vi "2foldstretch.vi"() -> ()   [LabVIEW 2012]
doc: "SciScan 1.2 160622"
uses:
  GFG/GFGImageRefsGet.vi
  <vilib>/vision/NI_Vision_Development_Module.lvlib
  GFG/GFG library.lvlib
panel:
  in  "stop":bool
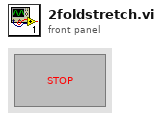
[diagram p1: front panel]
types:
  T1 = typedef "Image Type" = u32
  T2 = typedef "IMAQ Image.ctl" = refnum<image>
  T3 = cluster{"Channel 1 small":T2, "Channel 2 small":T2, "Channel 3 small":T2, "Channel 4 small":T2, "Channel 1 large":T2, "Channel 2 large":T2, "Channel 3 large":T2, "Channel 4 large":T2, "RGB overlay":T2, "ROI Image display":T2, "arb line scan display":T2, "Channel 5 large":T2}
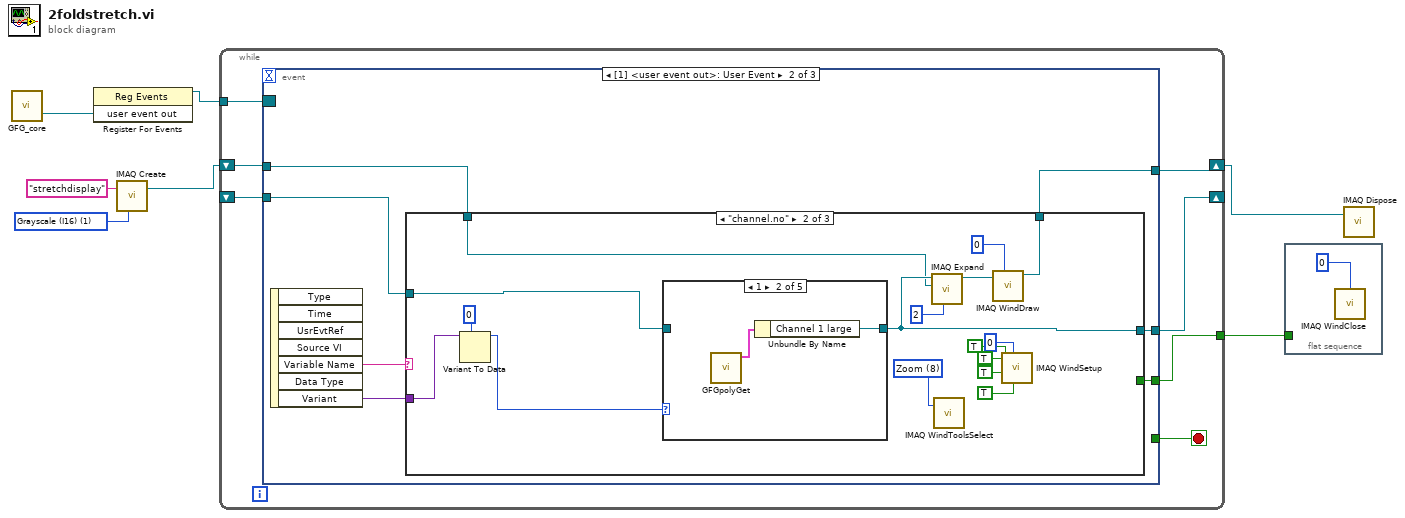
[diagram p0: block diagram]
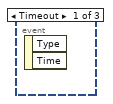
[diagram p2: hidden frame]
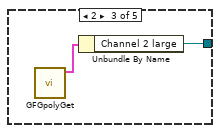
[diagram p5: hidden frame]
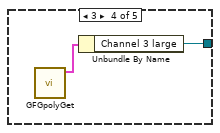
[diagram p6: hidden frame]
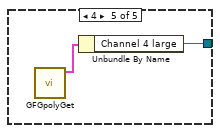
[diagram p7: hidden frame]
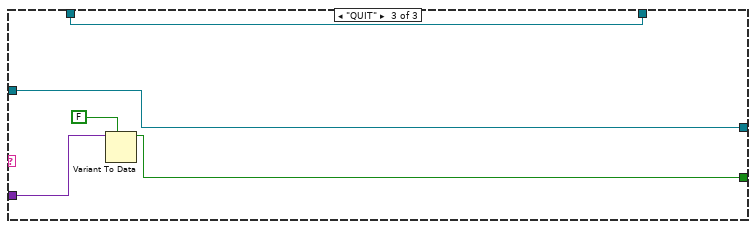
[diagram p8: hidden frame]
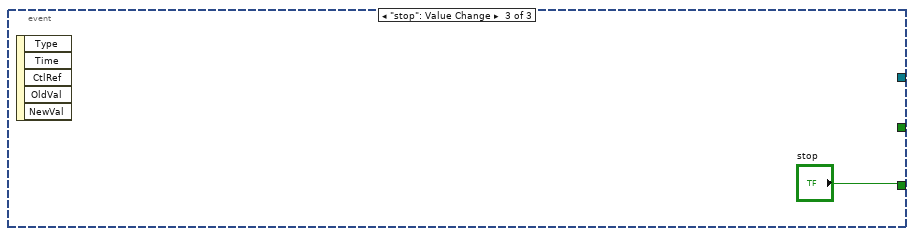
[diagram p9: hidden frame]
diagram:
  w2 = T1 1 items=["Grayscale (U8)", "Grayscale (I16)", "Grayscale (SGL)", "Complex (CSG)", "RGB (U32)", "HSL (U32)", "RGB (U64)", "Grayscale (U16)"] ("Image Type")
  n1 = call "GFG_core.vi"() -> ("user event out"=w6:refnum<user-event>)  [unwired: 13 in, 6 out]
  n2 = register-events(w6) -> (reference out=w7:refnum<event-registration>)  [unwired: 2 in, 1 out]
  n3 = call "IMAQ Create"("Image Name"="stretchdisplay", "Image Type"=w2) -> ("New Image"=w4:T2)  [unwired: 3 in, 1 out]
  n4 = while {
    tunnel: w7 -> [w14]
    shift-right: [w13] -> _
    shift-left: _ -> [w12]
    shift-right: [w11] -> w3
    shift-left: w4 -> [w10]
    tunnel: [w9] -> w1
    stop <- w8 stop-if-true
    n5 = event shown="[1] <user event out>: User Event" {
      selector: w14 -> [_ _ _]
      dyn-events: _ -> [_ _ _]
      timeout: _ -> [_ _ _]
      tunnel: [_ w19 _] -> w9
      tunnel: [_ w18 _] -> w13
      tunnel: w12 -> [_ w17 _]
      tunnel: w10 -> [_ w16 _]
      tunnel: [_ w15 _] -> w11
      tunnel: [_ _ "stop"] -> w8
      event Timeout {
        n6 = event-data() -> ()  [unwired: 1 in, 2 out]
      }
      event User Event {
        n7 = event-data() -> ("Variable Name"=w21:string, "Variant"=w20:variant)  [unwired: 1 in, 5 out]
        n8 = case shown="\"channel.no\"" w21 {
          tunnel: [_ _ w51] -> w19
          tunnel: w20 -> [_ w38 w53]
          tunnel: [w23 w36 w50] -> w18
          tunnel: w17 -> [w23 w37 w50]
          tunnel: w16 -> [w22 w35 w49]
          tunnel: [w22 w34 w49] -> w15
          frame "False", Default {
          }
          frame "channel.no" {
            w24 = u32 8 items=["No Selection", "Point", "Line", "Rectangle", "Oval", "Polygon", "Freehand Region", "Annulus", "Zoom", "Pan", "Broken Line", "Freehand Line", "Rotated Rectangle"] ("Tool (Point)")
            n9 = Variant To Data(type=0, Variant=w38) -> (data=w33:i32)  [unwired: 1 in, 1 out]
            n10 = case shown="1" w33 {
              tunnel: [w40 w41 w43 w45 w47] -> w36
              tunnel: w37 -> [w40 _ _ _ _]
              frame 0, Default {
              }
              frame 1 {
                n11 = call-poly "GFGpolyGet.vi"() -> ("Image Refs Out"=w42:T3)  [unwired: 10 in, 1 out]
                n12 = Unbundle By Name(w42) -> ("Channel 1 large"=w41:T2)
              }
              frame 2 {
                n13 = call-poly "GFGpolyGet.vi"() -> ("Image Refs Out"=w44:T3)  [unwired: 10 in, 1 out]
                n14 = Unbundle By Name(w44) -> ("Channel 2 large"=w43:T2)
              }
              frame 3 {
                n15 = call-poly "GFGpolyGet.vi"() -> ("Image Refs Out"=w46:T3)  [unwired: 10 in, 1 out]
                n16 = Unbundle By Name(w46) -> ("Channel 3 large"=w45:T2)
              }
              frame 4 {
                n17 = call-poly "GFGpolyGet.vi"() -> ("Image Refs Out"=w48:T3)  [unwired: 10 in, 1 out]
                n18 = Unbundle By Name(w48) -> ("Channel 4 large"=w47:T2)
              }
            }
            n19 = call "IMAQ Expand"("Y Duplication Step"=2, "Image Dst"=w35, "Image Src"=w36) -> ("Image Dst Out"=w32:T2)  [unwired: 7 in, 1 out]
            n20 = call "IMAQ WindToolsSelect"("Tool (Point)"=w24) -> ()  [unwired: 4 in, 2 out]
            n21 = call "IMAQ WindDraw"("Window Number (0...15)"=0, "Image"=w32) -> ("Image Out (duplicate)"=w34:T2)  [unwired: 8 in, 1 out]
            n22 = call "IMAQ WindSetup"("Window is floating? (No)"=TRUE, "Window Number (0...15)"=0, "Window has title bar? (Yes)"=TRUE, "Window can close? (Yes)"=TRUE, "Window can grow? (Yes)"=TRUE) -> ()  [unwired: 6 in, 1 out]
          }
          frame "QUIT" {
            n23 = Variant To Data(type=FALSE ("NewVal"), Variant=w53) -> (data=w51:bool)  [unwired: 1 in, 1 out]
          }
        }
      }
      event "stop": Value Change {
        n24 = event-data() -> ()  [unwired: 1 in, 5 out]
      }
    }
  }
  n25 = flat-sequence {
    tunnel: w1 -> [_]
    frame #0 {
      n26 = call "IMAQ WindClose"("Window Number (0...15)"=0) -> ()  [unwired: 5 in, 1 out]
    }
  }
  n27 = call "IMAQ Dispose"("Image"=w3) -> ()  [unwired: 5 in, 1 out]
